vi "Sub_Sharp_gerade.vi"(10 "gerade rechts":dbl, 11 "gerade links":dbl) -> (3 "grösser als 100?":bool)   [LabVIEW 2016]
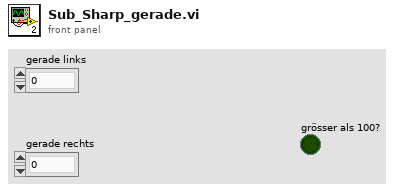
[diagram p1: front panel]
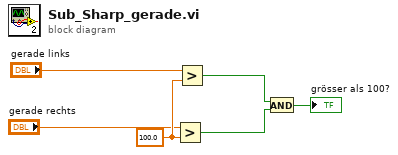
[diagram p0: block diagram]
diagram:
  w3 = 100.0 ("y")
  n1 = Greater?(x="gerade rechts", y=w3) -> (0:w5:bool)
  n2 = Greater?(x="gerade links", y=w3) -> (0:w4:bool)
  n3 = And(x=w4, y=w5) -> (x .and. y?=→"grösser als 100?":bool)
